vi "BBE com.vi"() -> ()   [LabVIEW 2016, in "bbe.lvlib"]
uses:
  bbe.lvlib
  <vilib>/Instr/_visa.llb/VISA Configure Serial Port (Instr).vi
panel:
  out "检测浓度":T1
  out "555 string":string
  out "553 string":string
  in  "布尔":bool
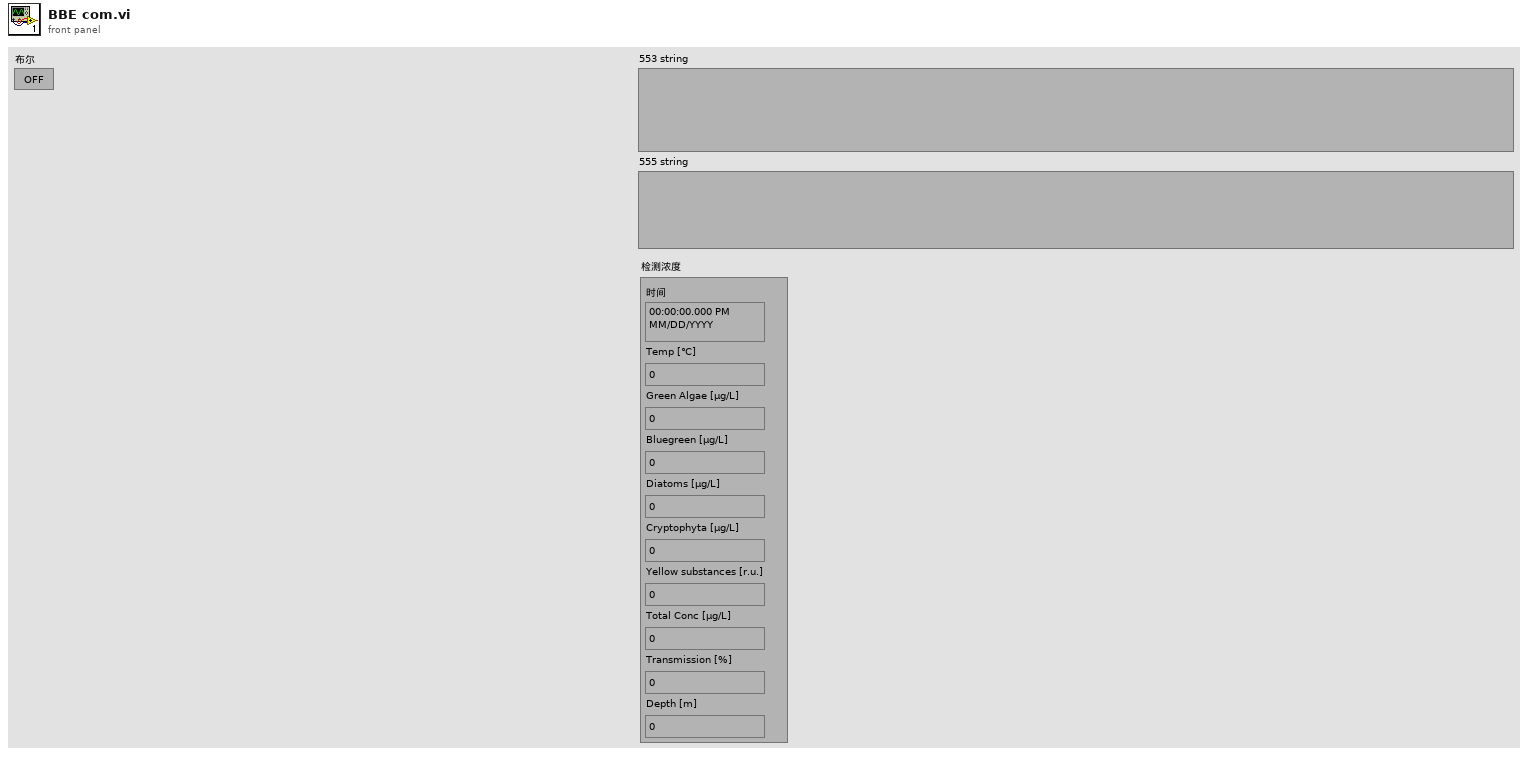
[diagram p1: front panel]
types:
  T1 = cluster{"时间":timestamp, "Temp [℃]":dbl, "Green Algae [μg/L]":dbl, "Bluegreen [μg/L]":dbl, "Diatoms [μg/L]":dbl, "Cryptophyta [μg/L]":dbl, "Yellow substances [r.u.]":dbl, "Total Conc [μg/L]":dbl, "Transmission [%]":dbl, "Depth [m]":dbl}
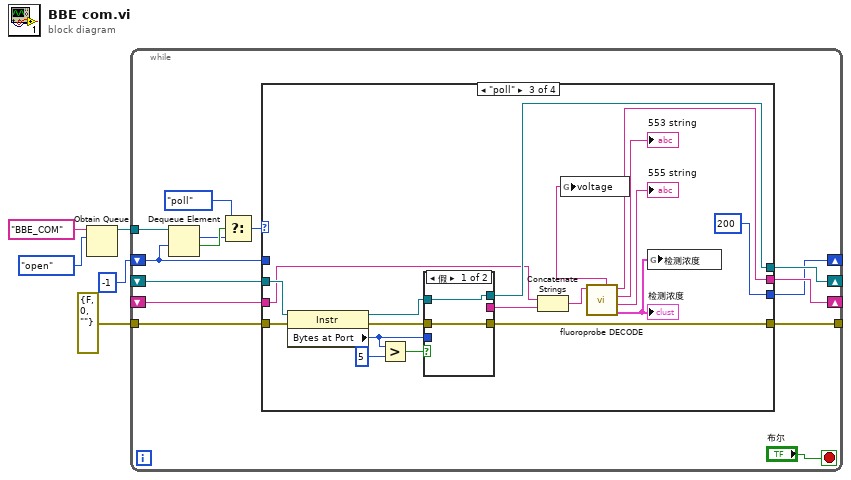
[diagram p0: block diagram]
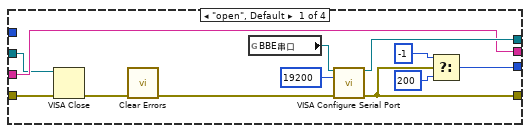
[diagram p2: hidden frame]
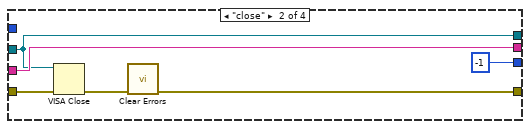
[diagram p3: hidden frame]
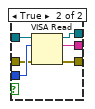
[diagram p4: hidden frame]
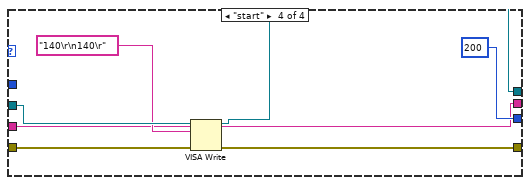
[diagram p5: hidden frame]
diagram:
  n1 = Obtain Queue(name (unnamed)="BBE_COM" ("名称（未命名）"), element data type=enum16{"open", "close", "poll", "start"}."open" ("枚举")) -> (queue out=w3:refnum<queue>)  [unwired: 3 in, 2 out]
  n2 = while {
    shift-right: [w17] -> _
    shift-left: _ -> [w19]
    shift-right: [w13] -> _
    shift-left: _ -> [w14]
    tunnel: w3 -> [w12]
    shift-right: [w11] -> _
    shift-left: -1 ("超时毫秒(-1)") -> [w10]
    tunnel: errorcluster {"status"=FALSE, "code"=0, "source"=""} ("error out") -> [w18]
    tunnel: [w16] -> _
    stop <- "布尔" stop-if-true
    n3 = Dequeue Element(queue=w12, timeout in ms (-1)=w10) -> (element=w8:enum16{"open", "close", "poll", "start"}, timed out?=w9:bool)  [unwired: 1 in, 2 out]
    n4 = Select(t=enum16{"open", "close", "poll", "start"}."poll" ("枚举"), s=w9, f=w8) -> (s? t:f=w7:enum16{"open", "close", "poll", "start"})
    n5 = case shown="\"poll\"" w7 {
      tunnel: w19 -> [w26 w33 w55 w70]
      tunnel: w18 -> [w27 w36 w54 w69]
      tunnel: [w30 w33 w50 w68] -> w17
      tunnel: [w23 w34 w49 w67] -> w16
      tunnel: w14 -> [w29 w37 w47 w64]
      tunnel: [w29 w37 w45 w64] -> w13
      tunnel: [w21 -1 ("超时毫秒(-1)") 200 ("超时毫秒(-1)") 200 ("超时毫秒(-1)")] -> w11
      tunnel: w10 -> [_ _ _ _]
      frame "open", Default {
        n6 = VISA Close(VISA resource name=w26, error in (no error)=w27) -> (error out=w25:errorcluster)
        n7 = call <vilib>:"Clear Errors.vi"("error in (no error)"=w25) -> ("error out"=w24:errorcluster)  [unwired: 5 in, 1 out]
        n8 = global read "过程变量.vi" "BBE串口"() -> (w28:refnum<visa-resource-name>)
        n9 = call-poly "VISA Configure Serial Port"("VISA resource name"=w28, "baud rate (9600)"=u32 19200, "error in (no error)"=w24) -> ("VISA resource name out"=w30:refnum<visa-resource-name>, "error out"=w23:errorcluster)  [unwired: 11 in]
        n10 = Select(t=-1 ("超时毫秒(-1)"), s=w23, f=200) -> (s? t:f=w21:i32)
      }
      frame "close" {
        n11 = VISA Close(VISA resource name=w33, error in (no error)=w36) -> (error out=w35:errorcluster)
        n12 = call <vilib>:"Clear Errors.vi"("error in (no error)"=w35) -> ("error out"=w34:errorcluster)  [unwired: 5 in, 1 out]
      }
      frame "poll" {
        n13 = property class="Instr"(reference=w55, error in=w54) -> (reference out=w53:refnum<visa-resource-name>, error out=w51:errorcluster, "Bytes at Port"=w40:u32)
        n14 = Greater?(x=w40, y=u32 5) -> (0:w52:bool)
        n15 = case shown="假" w52 {
          tunnel: w53 -> [w57 w63]
          tunnel: w40 -> [_ w62]
          tunnel: [w57 w61] -> w50
          tunnel: w51 -> [w56 w60]
          tunnel: [w56 w59] -> w49
          tunnel: [_ w58] -> w48
          frame False {
          }
          frame True {
            n16 = VISA Read(VISA resource name=w63, byte count=w62, error in (no error)=w60) -> (VISA resource name out=w61:refnum<visa-resource-name>, read buffer=w58:string, error out=w59:errorcluster)  [unwired: 1 out]
          }
        }
        n17 = Concatenate Strings(w47, w48) -> (w46:string)
        n18 = call "fluoroprobe DECODE.vi"("input string"=w46) -> ("检测浓度"=w41:T1, "555 string"=→"555 string":string, "553 string"=→"553 string":string, "output string"=w45:string, "voltage"=w38:string)  [unwired: 6 in]
        "检测浓度" <- w41
        n19 = global write "过程变量.vi" "voltage"(w38) -> ()
        n20 = global write "过程变量.vi" "检测浓度"(w41) -> ()
      }
      frame "start" {
        n21 = VISA Write(VISA resource name=w70, write buffer="140\r\n140\r" ("写入缓冲区"), error in (no error)=w69) -> (VISA resource name out=w68:refnum<visa-resource-name>, error out=w67:errorcluster)  [unwired: 1 out]
      }
    }
  }
